vi "StablizeDCV2.vi"(8 "Stability Criteria":dbl, 10 "DC":dbl, 11 "ArrayIn":dbl[](array[numeric]) format="%0.2f") -> (3 "Boolean":bool)   [LabVIEW 2014]
uses:
  <vilib>/Analysis/baseanly.llb/Mean (DBL).vi
  <vilib>/Analysis/NI_AALBase.lvlib
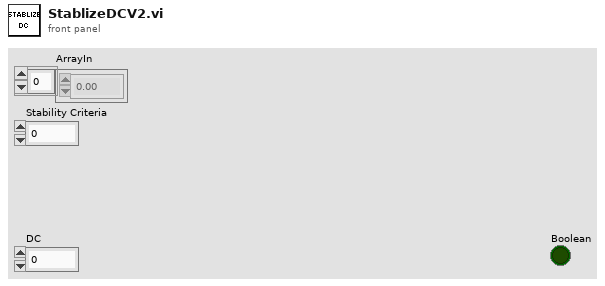
[diagram p1: front panel]
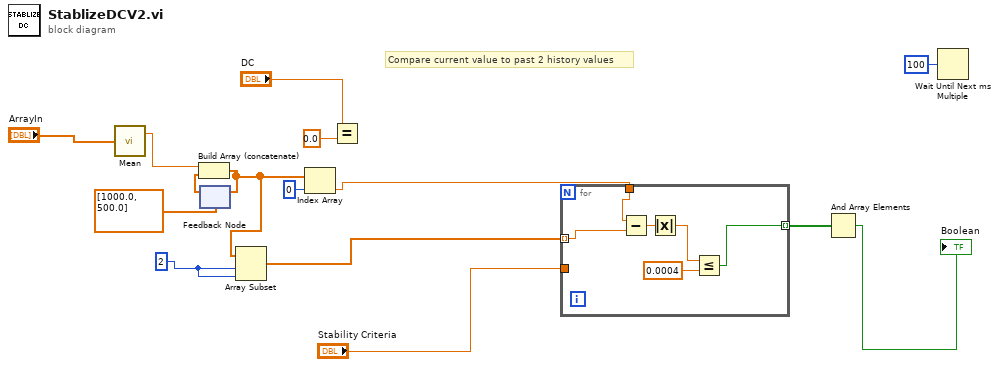
[diagram p0: block diagram]
diagram:
  w4 = 2 ("y")
  # "Compare current value to past 2 history values"
  n1 = call-poly <vilib>:"Mean.vi"("X"="ArrayIn") -> ("mean"=w9:dbl)  [unwired: 1 out]
  n2 = feedback #1(dbl[] [1000.0, 500.0]) -> (w10:dbl[])
  n3 = Build Array (concatenate)(w9, w10) -> (w13:dbl[])
  n4 = feedback-in #1(w13) -> ()
  n5 = Array Subset(array=w13, index=w4, length=w4) -> (w14:dbl[])
  n6 = Index Array(array=w13, index=0) -> (element=w12:dbl)
  n7 = Equal?(x="DC", y=0.0) -> ()  [unwired: 1 out]
  n8 = for {
    tunnel: w12 -> [w20]
    tunnel: w14 -> [w19] mode=indexing
    tunnel: "Stability Criteria" -> [_]
    tunnel: [w16] -> w1 mode=indexing
    n9 = Subtract(x=w20, y=w19) -> (x-y=w21:dbl)
    n10 = Absolute Value(x=w21) -> (abs(x)=w18:dbl)
    n11 = Less Or Equal?(x=w18, y=0.0004) -> (x <= y?=w16:bool)
  }
  n12 = And Array Elements(Boolean array=w1) -> (logical AND=→"Boolean":bool)
  n13 = Wait Until Next ms Multiple(millisecond multiple=u32 100) -> ()  [unwired: 1 out]
